vi "Shutdown.vi"(8 "error in (no error)":errorcluster, 11 "VeriStand Data Sharing Framework in":refnum<class "VeriStand Data Sharing Framework.lvclass">) -> (0 "error out":errorcluster, 3 "VeriStand Data Sharing Framework out":refnum<class "VeriStand Data Sharing Framework.lvclass">)   [LabVIEW 2017, in "Data Sharing Custom Device Engine.lvlib" / "VeriStand Data Sharing Framework.lvclass"]
uses:
  VeriStand Data Sharing Framework.lvclass
  Builds/Data Sharing Framework/Current/Core/DSF Core.lvlibp/Engine/Classes/Framework/Framework.lvclass
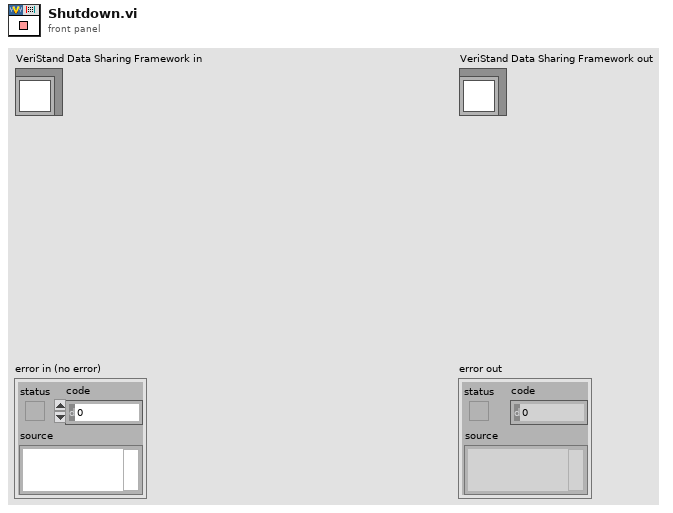
[diagram p1: front panel]
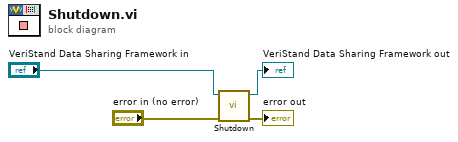
[diagram p0: block diagram]
diagram:
  n1 = call-parent "Shutdown.vi"("error in (no error)"="error in (no error)", "Framework in"="VeriStand Data Sharing Framework in") -> ("error out"=→"error out":errorcluster, "Framework out"=→"VeriStand Data Sharing Framework out":refnum<class "VeriStand Data Sharing Framework.lvclass">)  [unwired: 8 in]
